vi "AMX-CCD 自动处理图像 - 副本.vi"(8 "error in (no error)":errorcluster caption="错误输入（无错误）") -> (0 "error out":errorcluster caption="错误输出", 3 "Image Out":T4(plugin-control), 11 "Image In":T4(plugin-control))   [LabVIEW 2017]
panel:
  in  "UI电源线正面标签1参数 2":T2={"Rectangle"={"Left"=0, "Top"=0, "Right"=0, "Bottom"=0, "Rotation"=0.0}, "Angle (degrees) (Geometry 1)"=90.0, "中心位置"={"Cent X"=273.0, "Cent Y"=255.0, "半径"=300.0}, "long"=300.0, "abgek"=0.0, "Color"=16711680, "left threshold"=0.0, "Rectangle right"={"Left"=0, "Top"=0, "Right"=0, "Bottom"=0, "Rotation"=0.0}, "long right"=300.0, "abgek right"=0.0, "Color 2"=16711680, "right threshold"=0.0, "left"=0.0, "right"=0.0} {"Rectangle right"."Rotation" format="%.2f"; "Rectangle right"."Left" scale=0.0..1024.0; "Rectangle right"."Right" scale=0.0..1024.0; "Rectangle"."Rotation" format="%.2f"; "Rectangle"."Left" scale=0.0..1024.0; "Rectangle"."Right" scale=0.0..1024.0}
  in  "电源线正面标签1基础参数":T3={"IsNorImage"=TRUE, "Exposure Values"=100289, "ImagePath"=path "C:/Users/hedongpo/Desktop/514-hdp/Alignment Assemble System/Test Picture/B/3.bmp"} caption="参数界面" {"Exposure Values" scale=0.0..200000.0}
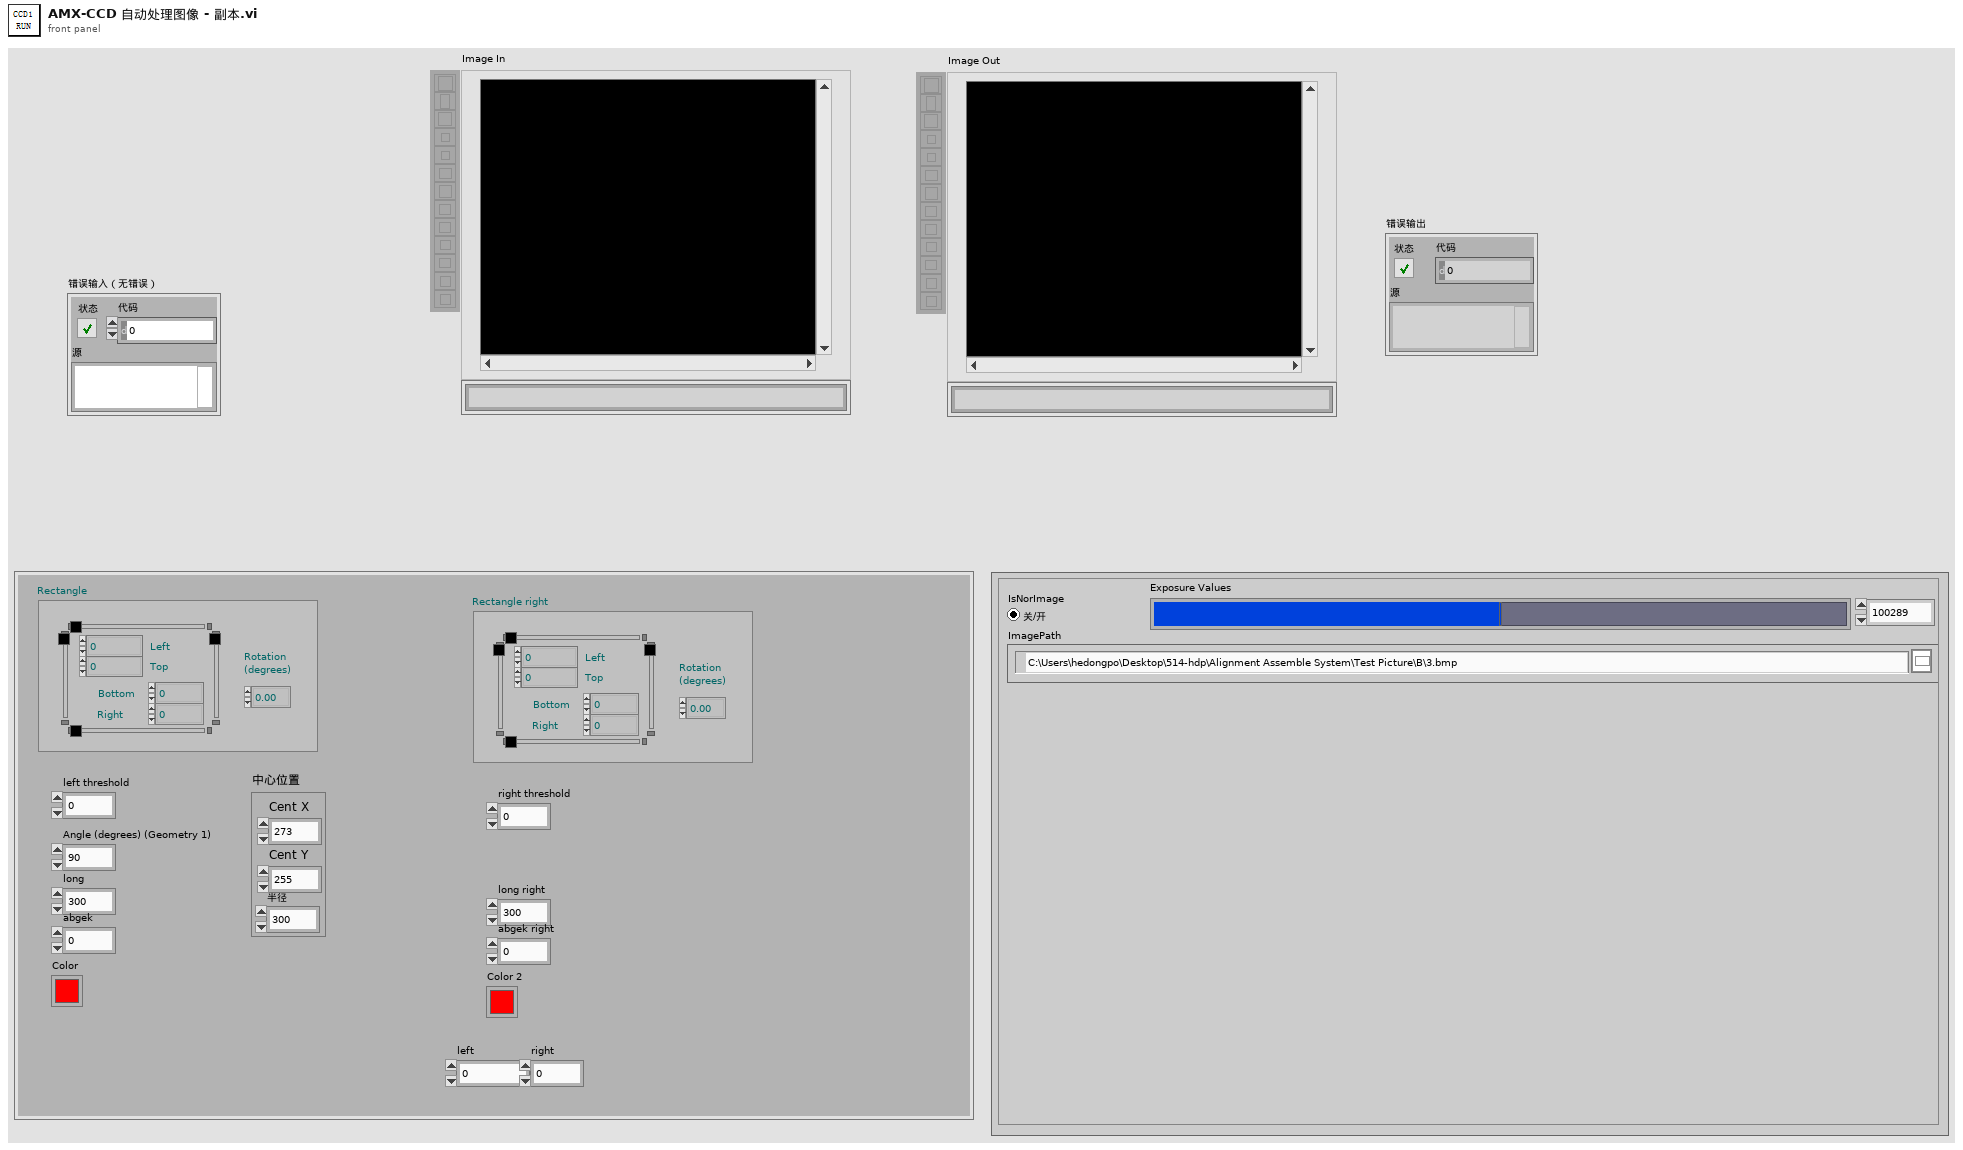
[diagram p1: front panel]
types:
  T1 = typedef "IMAQ Rectangle" = cluster{"Left":i32, "Top":i32, "Right":i32, "Bottom":i32, "Rotation":dbl}
  T2 = cluster{"Rectangle":T1, "Angle (degrees) (Geometry 1)":sgl, "中心位置":cluster{"Cent X":dbl, "Cent Y":dbl, "半径":dbl}, "long":sgl, "abgek":dbl, "Color":u32, "left threshold":dbl, "Rectangle right":T1, "long right":sgl, "abgek right":dbl, "Color 2":u32, "right threshold":dbl, "left":dbl, "right":dbl}
  T3 = cluster{"IsNorImage":bool, "Exposure Values":u32, "ImagePath":path}
  T4 = typedef "IMAQ Image.ctl" = refnum<image>
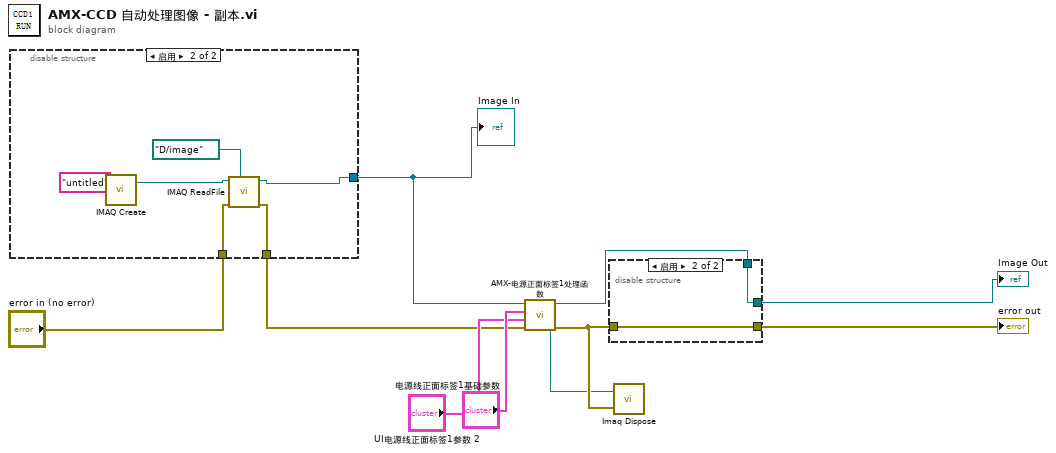
[diagram p0: block diagram]
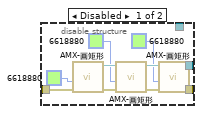
[diagram p3: hidden frame]
diagram:
  n1 = disable-structure shown="启用" {
    disable-tunnel: [_ w15] -> w1
    disable-tunnel: [_ w12] -> w3
    disable-tunnel: "error in (no error)" -> [_ w11]
    frame Disabled {
    }
    frame Enabled {
      n2 = call "IMAQ Create"("Image Name"="untitled") -> ("New Image"=w14:T4)  [unwired: 4 in, 1 out]
      n3 = call "IMAQ ReadFile"("File Path"=path "D:/image", "error in (no error)"=w11, "Image"=w14) -> ("error out"=w12:errorcluster, "Image Out"=w15:T4)  [unwired: 4 in, 3 out]
    }
  }
  "Image In" <- w1
  n4 = call "AMX-电源正面标签1处理函数.vi"("error in (no error)"=w3, "UI电源线正面标签1参数 2"="UI电源线正面标签1参数 2", "电源线正面标签1基础参数"="电源线正面标签1基础参数", "Image in"=w1) -> ("error out"=w7:errorcluster, "Image out"=w6:T4)  [unwired: 6 in]
  n5 = disable-structure shown="启用" {
    disable-tunnel: w7 -> [w25 w27]
    disable-tunnel: [w17 w26] -> w9
    disable-tunnel: [w16 w27] -> w8
    disable-tunnel: w6 -> [_ w26]
    frame Disabled {
      n6 = call "AMX-画矩形.vi"("error in (no error)"=w25, "Color"=u32 6618880) -> ("error out"=w21:errorcluster, "Image Out"=w23:T4)  [unwired: 8 in]
      n7 = call "AMX-画矩形.vi"("error in (no error)"=w21, "Color"=u32 6618880, "Image In"=w23) -> ("error out"=w18:errorcluster, "Image Out"=w20:T4)  [unwired: 7 in]
      n8 = call "AMX-画矩形.vi"("error in (no error)"=w18, "Color"=u32 6618880, "Image In"=w20) -> ("error out"=w16:errorcluster, "Image Out"=w17:T4)  [unwired: 7 in]
    }
    frame Enabled {
    }
  }
  "error out" <- w8
  "Image Out" <- w9
  n9 = call "Imaq Dispose"("Image"=w6, "error in (no error)"=w7) -> ()  [unwired: 4 in, 1 out]
